vi "Core.vi"(6 "Show FP?":bool, 8 "error in (no error)":errorcluster, 11 "Sim DiscreteIO in":refnum<class "Sim DiscreteIO.lvclass">) -> (0 "error out":errorcluster, 3 "Sim DiscreteIO out":refnum<class "Sim DiscreteIO.lvclass">)   [LabVIEW 2021, in "Sim DiscreteIO.lvclass"]
uses:
  Sim DiscreteIO.lvclass
  <userlib>/S2 Labs/Module Framework/Modules/Base/Module.lvclass
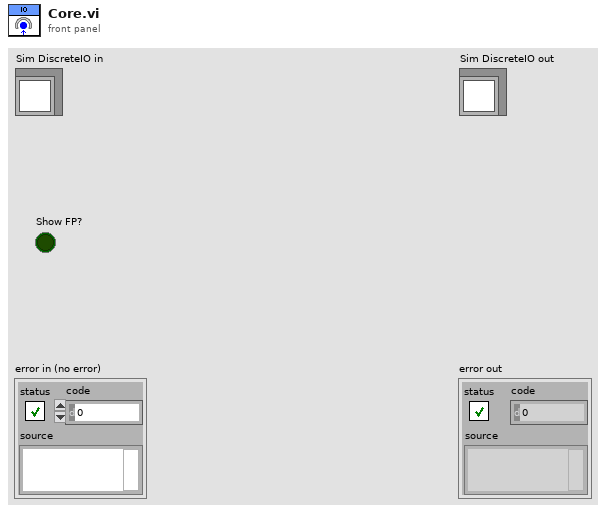
[diagram p1: front panel]
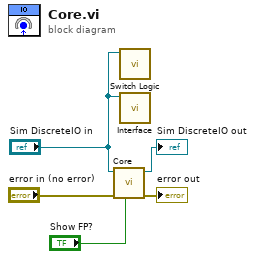
[diagram p0: block diagram]
diagram:
  n1 = call-parent "Core.vi"("Show FP?"="Show FP?", "error in (no error)"="error in (no error)", "Module in"="Sim DiscreteIO in") -> ("error out"=→"error out":errorcluster, "Module out"=→"Sim DiscreteIO out":refnum<class "Sim DiscreteIO.lvclass">)  [unwired: 7 in]
  n2 = call "Switch Logic.vi"("Sim DiscreteIO in"="Sim DiscreteIO in") -> ()  [unwired: 10 in, 1 out]
  n3 = call "Interface.vi"("Sim DiscreteIO in"="Sim DiscreteIO in") -> ()  [unwired: 10 in, 1 out]
